vi "Set Params.vi"(8 "error in (no error)":errorcluster, 11 "Fluke Calibrator in":refnum<class "Fluke Calibrator.lvclass">) -> (0 "error out":errorcluster, 3 "Fluke Calibrator out":refnum<class "Fluke Calibrator.lvclass">)   [LabVIEW 2012, in "Fluke Calibrator.lvclass"]
uses:
  Fluke Calibrator.lvclass
  Fluke Calibrator.lvclass/Fluke Calibrator.ctl
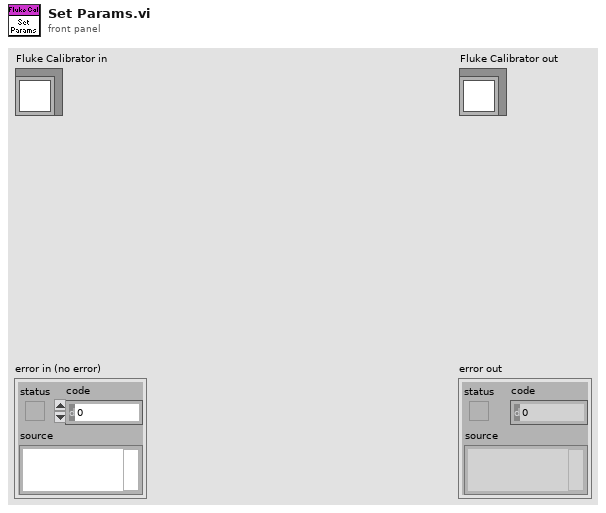
[diagram p1: front panel]
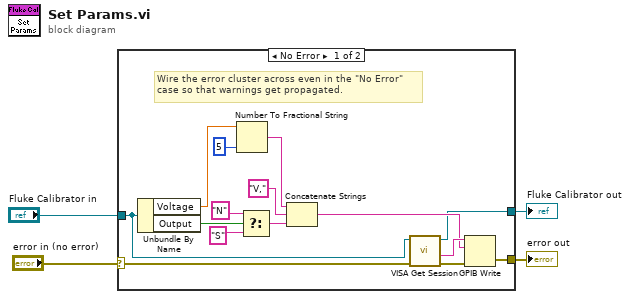
[diagram p0: block diagram]
diagram:
  n1 = case shown="No Error" "error in (no error)" {
    selector: "error in (no error)" -> [w19 w21]
    tunnel: [w13 w21] -> w3
    tunnel: [w6 w20] -> w1
    tunnel: "Fluke Calibrator in" -> [w7 w20]
    frame No Error {
      # "Wire the error cluster across even in the \"No Error\"\ncase so that warnings get propagated."
      n2 = Unbundle By Name(w7) -> ("Voltage"=w12:dbl, "Output"=w11:bool)
      n3 = Number To Fractional String(number=w12, precision (6)=i16 5) -> (F-format string=w16:string)  [unwired: 2 in]
      n4 = Select(t="N", s=w11, f="S") -> (s? t:f=w8:string)
      n5 = Concatenate Strings(w16, "V,", w8) -> (w14:string)
      n6 = call-dynamic "VISA Get Session.vi"("error in (no error)"=w19, "Instrument.lvclass in"=w7) -> ("error out"=w18:errorcluster, "GPIB string"=w17:string, "Instrument.lvclass out"=w6:refnum<class "Fluke Calibrator.lvclass">)  [unwired: 6 in, 1 out]
      n7 = GPIB Write(0:w17, 1:w14, 3:w18) -> (6:w13:errorcluster)  [unwired: 2 in, 1 out]
    }
    frame Error {
    }
  }
  "error out" <- w3
  "Fluke Calibrator out" <- w1
